vi "Close Bus Monitor.vi"(8 "error in (no error)":errorcluster, 11 "IBusMonitor In":refnum<class "IBusMonitor.lvclass">) -> (3 "IBusMonitor Out":refnum<class "IBusMonitor.lvclass">)   [LabVIEW 2020, in "MonitoredMediator.lvlib" / "IBusMonitor.lvclass"]
doc: "抽象方法\n关闭总线监视器"
uses:
  IBusMonitor.lvclass
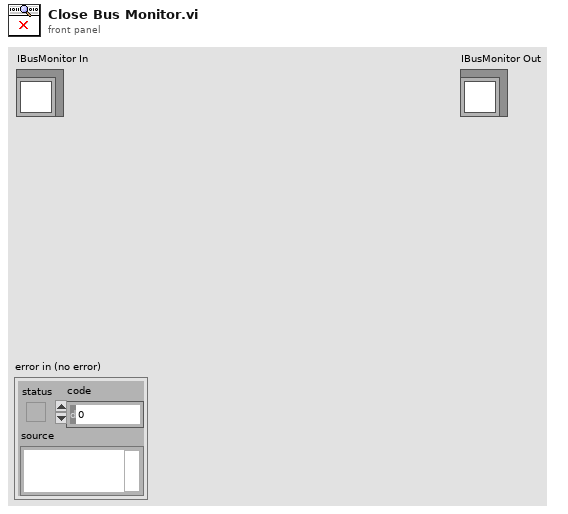
[diagram p1: front panel]
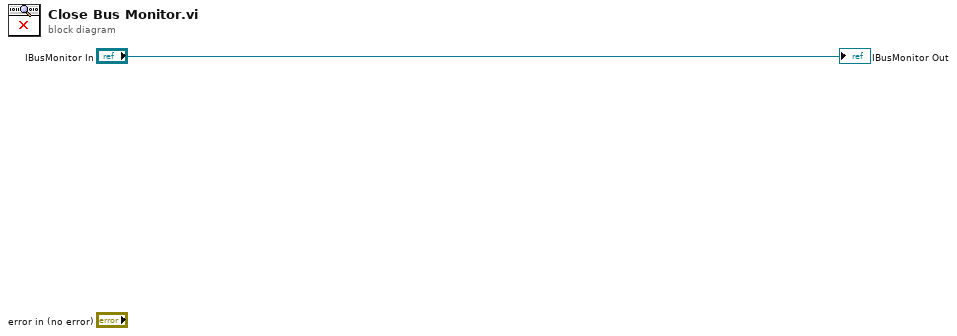
[diagram p0: block diagram]
diagram:
  "IBusMonitor Out" <- "IBusMonitor In"
